vi "Close MeasurementLink Session.vi"(8 "error in":errorcluster, 9 "close session behavior":T1, 10 "session in":variant, 11 "instrument in":refnum<class "Instrument.lvclass">) -> (0 "error out":errorcluster)   [LabVIEW 2020, in "MeasurementLink niDCPower.lvlib" / "Instrument.lvclass"]
doc: "Closes the local NI-DCPower session. If the <b>close session behavior</b> input is <b>Close Session</b>, the session on the NI gRPC Device Server will be closed. If the <b>close session behavior</b> input is <b>Detach Session</b>, the session on the NI gRPC Device Server will remain open."
uses:
  Instrument.lvclass
  MeasurementLink Instrument/IInstrument/Close Session Behavior.ctl
  Instrument.lvclass/Instrument.ctl
  MeasurementLink Instrument/IInstrument/IInstrument.lvclass
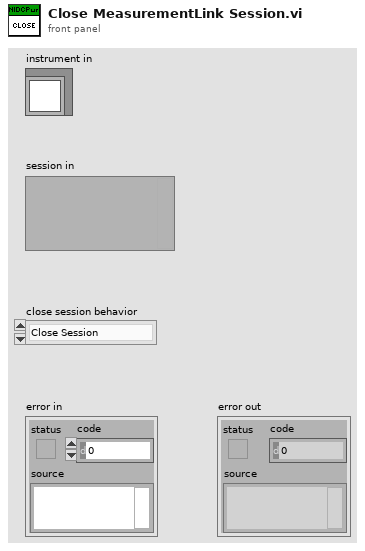
[diagram p1: front panel]
types:
  T1 = typedef "MeasurementLink Instrument.lvlib/IInstrument.lvclass/Close Session Behavior.ctl" = enum16{"Close Session", "Detach Session"}
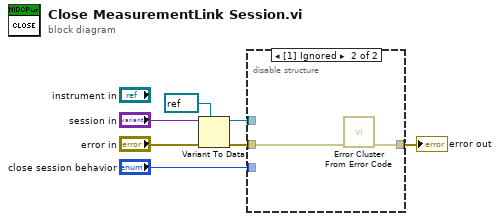
[diagram p0: block diagram]
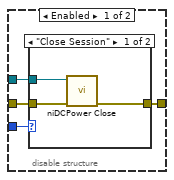
[diagram p2: hidden frame]
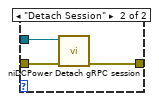
[diagram p3: hidden frame]
diagram:
  n1 = Variant To Data(error in="error in", type=refnum<k15> refnum ("instrument handle"), Variant="session in") -> (data=w2:refnum<k15>, error out=w3:errorcluster)
  n2 = disable-structure shown="[1] Ignored" {
    disable-tunnel: "close session behavior" -> [w11 _]
    disable-tunnel: w3 -> [w10 w18]
    disable-tunnel: w2 -> [w9 _]
    disable-tunnel: [w8 w19] -> w1
    frame Enabled {
      n3 = case shown="\"Close Session\"" w11 {
        tunnel: w10 -> [w14 w17]
        tunnel: w9 -> [w13 w16]
        tunnel: [w12 w15] -> w8
        frame "Close Session" {
          n4 = call <instrlib>:"niDCPower Close.vi"("error in (no error)"=w14, "instrument handle"=w13) -> ("error out"=w12:errorcluster)  [unwired: 9 in]
        }
        frame "Detach Session" {
          n5 = call <instrlib>:"niDCPower Detach gRPC session.vi"("error in (no error)"=w17, "instrument handle"=w16) -> ("error out"=w15:errorcluster)  [unwired: 9 in]
        }
      }
    }
    frame Disabled {
      n6 = call <vilib>:"Error Cluster From Error Code.vi"("error in (no error)"=w18) -> ("error out"=w19:errorcluster)  [unwired: 8 in]
    }
  }
  "error out" <- w1
